vi "make xy voltage map.vi"() -> ()   [LabVIEW 2012]
uses:
  GFG/GFGnumericGet.vi
  GFG/GFGbooleanGet.vi
  GFG/GFG library.lvlib
panel:
  out "x voltage (after applying shift for Start.Delay)":T1(plugin-control)
  out "y voltage (after applying shift for Start.Delay)":T1(plugin-control)
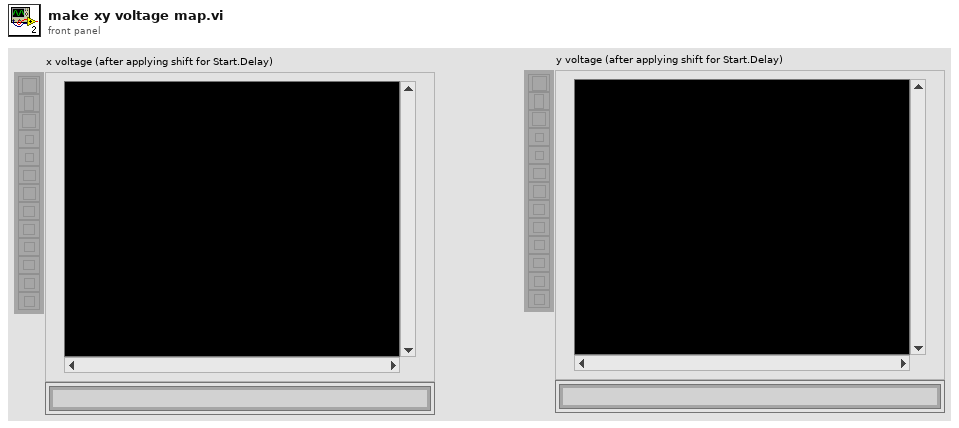
[diagram p1: front panel]
types:
  T1 = typedef "IMAQ Image.ctl" = refnum<image>
  T2 = cluster{"xyvoltagefor2frames":dbl[][][], "x.pixels":dbl, "nomin.x.pixels":dbl, "y.pixels":dbl, "fill.fraction":dbl, "x.bidirectional":bool, "y.bidirectional":bool}
  T3 = typedef "Image Type" = u32
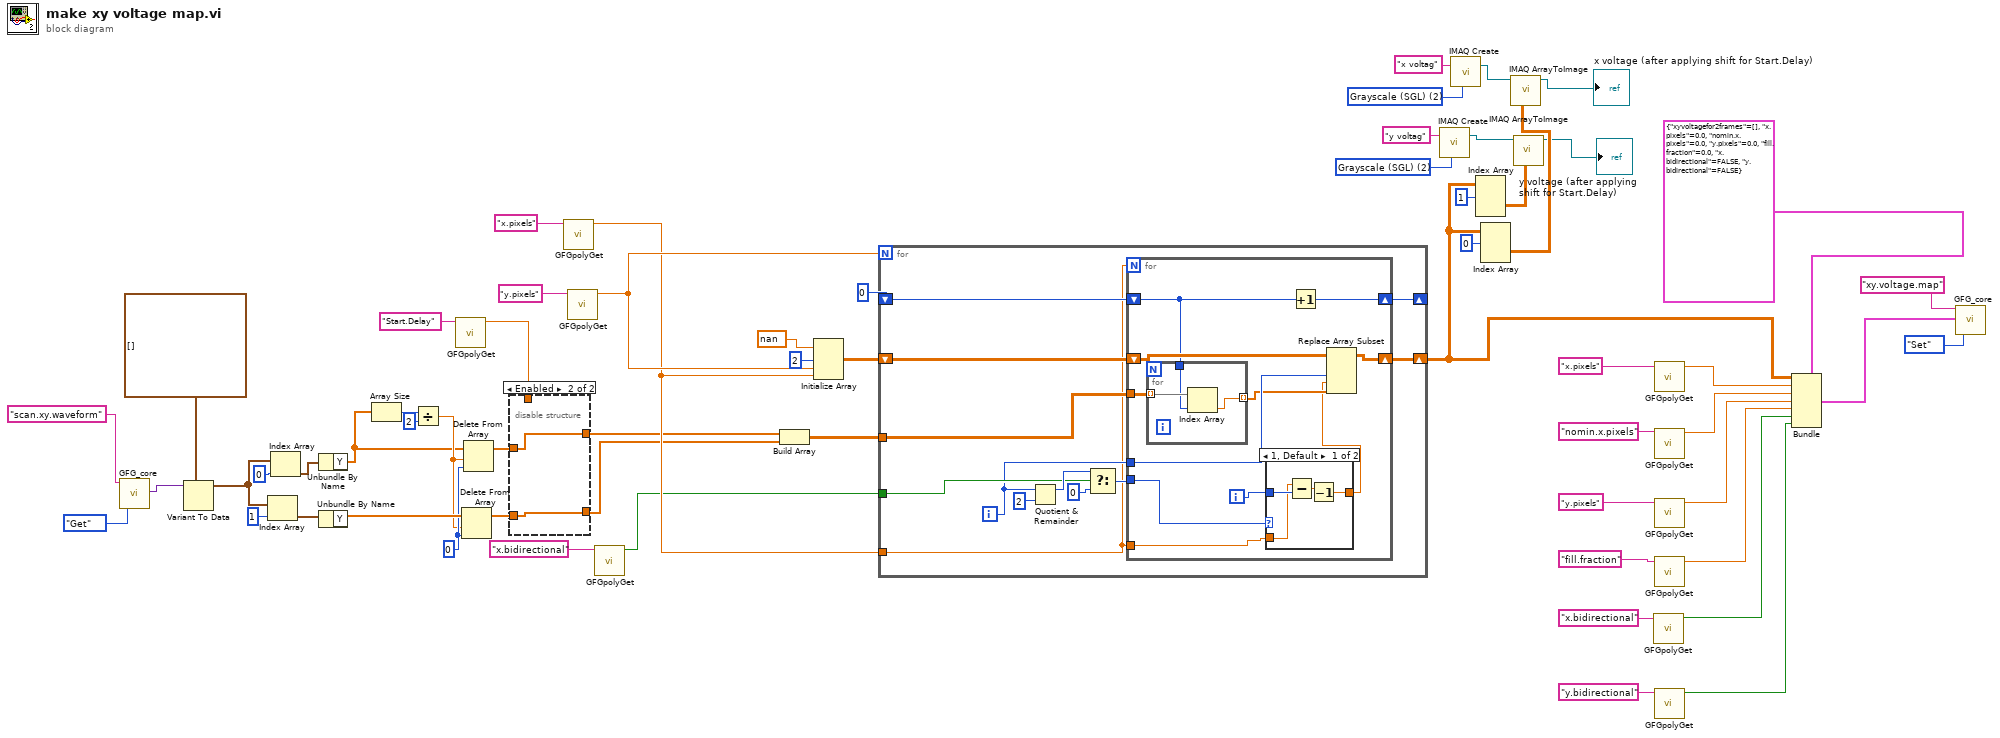
[diagram p0: block diagram]
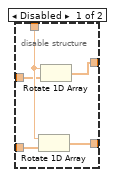
[diagram p2: hidden frame]
diagram:
  w24 = T3 2 items=["Grayscale (U8)", "Grayscale (I16)", "Grayscale (SGL)", "Complex (CSG)", "RGB (U32)", "HSL (U32)", "RGB (U64)", "Grayscale (U16)"] ("Image Type")
  w27 = T3 2 items=["Grayscale (U8)", "Grayscale (I16)", "Grayscale (SGL)", "Complex (CSG)", "RGB (U32)", "HSL (U32)", "RGB (U64)", "Grayscale (U16)"] ("Image Type")
  w41 = 0 ("index")
  n1 = call "GFG_core.vi"("Variable Name in"="scan.xy.waveform", "Action"=enum16{"Init", "Set", "Get"}."Get") -> ("Variant Out"=w30:variant)  [unwired: 11 in, 6 out]
  n2 = Variant To Data(type=waveform(dbl)[] [] ("frame scan geometry out"), Variant=w30) -> (data=w32:waveform(dbl)[])  [unwired: 1 in, 1 out]
  n3 = Index Array(array=w32, index=1) -> (element=w36:waveform(dbl))
  n4 = Index Array(array=w32, index=0) -> (element=w35:waveform(dbl))
  n5 = Unbundle By Name(w35) -> ("Y"=w39:dbl[])
  n6 = Unbundle By Name(w36) -> ("Y"=w42:dbl[])
  n7 = Array Size(array=w39) -> (size(s)=w37:i32)
  n8 = Divide(x=w37, y=2) -> (x/y=w40:dbl)
  n9 = call-poly "GFGpolyGet.vi"("Variable Name in"="Start.Delay") -> ("Numeric"=w46:dbl)  [unwired: 9 in, 1 out]
  n10 = Delete From Array(array=w42, length=w40, index=w41) -> (array with subset deleted=w45:dbl[])  [unwired: 1 out]
  n11 = Delete From Array(array=w39, length=w40, index=w41) -> (array with subset deleted=w43:dbl[])  [unwired: 1 out]
  n12 = disable-structure shown="Enabled" {
    disable-tunnel: [w66 w67] -> w55
    disable-tunnel: [w65 w68] -> w54
    disable-tunnel: w46 -> [w64 _]
    disable-tunnel: w45 -> [w63 w67]
    disable-tunnel: w43 -> [w62 w68]
    frame Disabled {
      n13 = Rotate 1D Array(1:w63, 2:w64) -> (0:w66:dbl[])
      n14 = Rotate 1D Array(1:w62, 2:w64) -> (0:w65:dbl[])
    }
    frame Enabled {
    }
  }
  n15 = call-poly "GFGpolyGet.vi"("Variable Name in"="x.pixels" ("Tag in")) -> ("Numeric"=w57:dbl)  [unwired: 9 in, 1 out]
  n16 = call-poly "GFGpolyGet.vi"("Variable Name in"="y.pixels" ("Tag in")) -> ("Numeric"=w58:dbl)  [unwired: 9 in, 1 out]
  n17 = call-poly "GFGpolyGet.vi"("Variable Name in"="x.bidirectional" ("Tag in")) -> ("Boolean"=w50:bool)  [unwired: 10 in]
  n18 = Build Array(w54, w55) -> (w56:dbl[][])
  n19 = Initialize Array(nan ("element"), 2 ("dimension size"), w58, w57) -> (w52:dbl[][][])
  n20 = for {
    N: w58 -> [_]
    tunnel: w57 -> [w70]
    tunnel: w50 -> [w76]
    shift-right: [w69] -> w5
    shift-left: w52 -> [w73]
    shift-right: [w74] -> _
    shift-left: 0 ("y") -> [w75]
    tunnel: w56 -> [w71]
    i -> [w72]
    n21 = Quotient & Remainder(x=w72, y=2) -> (x-y*floor(x/y)=w80:i32)  [unwired: 1 out]
    n22 = Select(t=w80, s=w76, f=0) -> (s? t:f=w77:i32)
    n23 = for {
      N: w70 -> [_]
      tunnel: w77 -> [w91]
      shift-right: [w90] -> w74
      shift-left: w75 -> [w83]
      shift-right: [w87] -> w69
      shift-left: w73 -> [w88]
      tunnel: w72 -> [w86]
      tunnel: w71 -> [w85]
      tunnel: w70 -> [w81]
      i -> [w89]
      n24 = for {
        tunnel: w85 -> [w94] mode=indexing
        tunnel: w83 -> [w93]
        tunnel: [w92] -> w84 mode=indexing
        n25 = Index Array(array=w94, index=w93) -> (element=w92:dbl)
      }
      n26 = case shown="1, Default" w91 {
        tunnel: w89 -> [w98 w99]
        tunnel: [w95 w99] -> w82
        tunnel: w81 -> [w97 _]
        frame 1, Default {
          n27 = Subtract(x=w97, y=w98) -> (x-y=w96:dbl)
          n28 = Decrement(x=w96) -> (x-1=w95:dbl)
        }
        frame 0 {
        }
      }
      n29 = Increment(x=w83) -> (x+1=w90:i32)
      n30 = Replace Array Subset(array=w88, new element=w84, index (dim 1)=w86, index (dim 2)=w82) -> (w87:dbl[][][])  [unwired: 1 in]
    }
  }
  n31 = call "IMAQ Create"("Image Name"="y voltag", "Image Type"=w24) -> ("New Image"=w22:T1)  [unwired: 3 in, 1 out]
  n32 = call "IMAQ Create"("Image Name"="x voltag", "Image Type"=w27) -> ("New Image"=w23:T1)  [unwired: 3 in, 1 out]
  n33 = Index Array(array=w5, index (dim 0)=1 ("index (page)")) -> (element=w17:dbl[][])  [unwired: 2 in]
  n34 = Index Array(array=w5, index (dim 0)=0 ("index (page)")) -> (element=w20:dbl[][])  [unwired: 2 in]
  n35 = call "IMAQ ArrayToImage"("Image Pixels (Float)"=w20, "Image"=w23) -> ("Image Out"=→"x voltage (after applying shift for Start.Delay)":T1)  [unwired: 8 in, 1 out]
  n36 = call "IMAQ ArrayToImage"("Image Pixels (Float)"=w17, "Image"=w22) -> ("Image Out"=→"y voltage (after applying shift for Start.Delay)":T1)  [unwired: 8 in, 1 out]
  n37 = call-poly "GFGpolyGet.vi"("Variable Name in"="x.bidirectional" ("Tag in")) -> ("Boolean"=w6:bool)  [unwired: 10 in]
  n38 = call-poly "GFGpolyGet.vi"("Variable Name in"="x.pixels" ("Tag in")) -> ("Numeric"=w10:dbl)  [unwired: 9 in, 1 out]
  n39 = call-poly "GFGpolyGet.vi"("Variable Name in"="nomin.x.pixels") -> ("Numeric"=w9:dbl)  [unwired: 9 in, 1 out]
  n40 = call-poly "GFGpolyGet.vi"("Variable Name in"="y.pixels" ("Tag in")) -> ("Numeric"=w8:dbl)  [unwired: 9 in, 1 out]
  n41 = call-poly "GFGpolyGet.vi"("Variable Name in"="fill.fraction") -> ("Numeric"=w7:dbl)  [unwired: 9 in, 1 out]
  n42 = call-poly "GFGpolyGet.vi"("Variable Name in"="y.bidirectional" ("Tag in")) -> ("Boolean"=w1:bool)  [unwired: 10 in]
  n43 = Bundle(cluster=T2 {"xyvoltagefor2frames"=[], "x.pixels"=0.0, "nomin.x.pixels"=0.0, "y.pixels"=0.0, "fill.fraction"=0.0, "x.bidirectional"=FALSE, "y.bidirectional"=FALSE} ("output cluster"), "xyvoltagefor2frames"=w5, "x.pixels"=w10, "nomin.x.pixels"=w9, "y.pixels"=w8, "fill.fraction"=w7, "x.bidirectional"=w6, "y.bidirectional"=w1) -> (w4:T2)
  n44 = call "GFG_core.vi"("Variable Name in"="xy.voltage.map", "Variant in"=w4, "Action"=enum16{"Init", "Set", "Get"}."Set") -> ()  [unwired: 10 in, 7 out]
